vi "ICM Play Back.vi"() -> ()   [LabVIEW 2024]
doc: "OSDS Simulator.vi\n\n This VI is used to produce simulated data streams, either by playing back files recorded with the OSDS Recorder.vi or by creating simulated data consistent with an OSDS definition file.\n\nOCC Streaming Data System Version 1.2.1\nMay, 2015 Original Code Consulting David Thomson\n www.originalcode.com\n\nOSDS is licensed under the Creative Commons Attribution-Share Alike 3.0 license (http://creativecommons.org/). Derivative and commercial works incorporating OSDS are allowed, as long as changes you make are made available to the community at large. Please submit improvements as well as new OSDS Format Files and OSDS Stream Files to support@originalcode.com"
uses:
  ICM Simulator State.ctl
  MICAS-X/Resources/OSDS/OSDS Subvis/OSDS Simulated Channel.ctl
  Bus/Bus.lvclass
  SubVIs/ICM Editor Stop.vi
  Instance           1 22Saved   OSDS Simulator .vi
panel:
  in  "stop":bool
  in  "Tab":enum32{"Setup", "Play Back"}(tab)
  in  "Play Back":bool
  in  "Load":bool
  in  "Loop":bool
  out "Stream File":path
  out "Data":T1(array[cluster]) {"Time Stamp" format="%<%H:%M:%S%1u>t"}
  in  "Display Style":enum16{"Normal", "Codes", "Password", "Hex"}(ring)
  in  "Clear Error":bool
  in  "Stop Streaming":bool
  out "Error":errorcluster
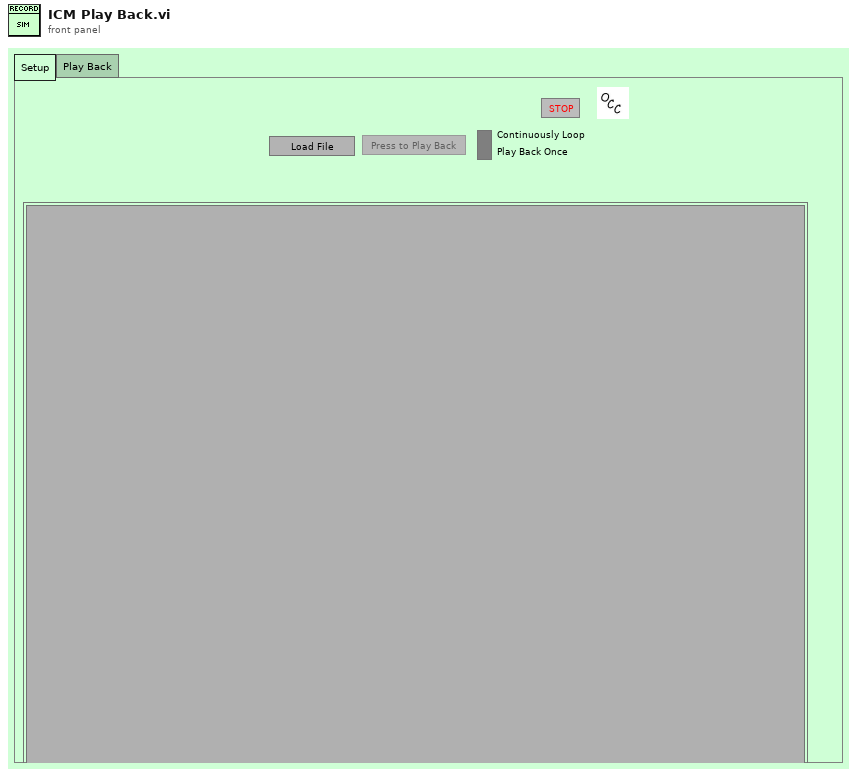
[diagram p1: front panel]
types:
  T1 = cluster{"Time Stamp":dbl, "Length":i32, "Data":string}[]
  T2 = typedef "ICM Simulator State.ctl" = enum16{"Initialize", "Wait", "Open File", "Open ICM", "Write String", "Stop Streaming", "Stop"}
  T3 = enum32{"invalid app kind", "Development System", "Run Time System", "Student Edition", "Embedded LabVIEW", "Evaluation", "Custom"}
  T4 = enum8{"Enabled", "Disabled", "Disabled and Grayed Out"}
  T5 = typedef "OSDS Simulated Channel.ctl" = enum16{"Zero", "Second", "Minute", "Hour", "Day", "Month", "Year", "Day of Year", "Sec of Day", "Latitude", "Longitude", "Altitude", "Nan", "Count", "Random", "One"}
  T6 = cluster{"Streaming?":bool, "Start Time":timestamp, "Current Position":i32, "Handle Out":variant, "Simulated Channels":T5[]}
  T7 = cluster{"Time Stamp":dbl, "Length":i32, "Data":string}
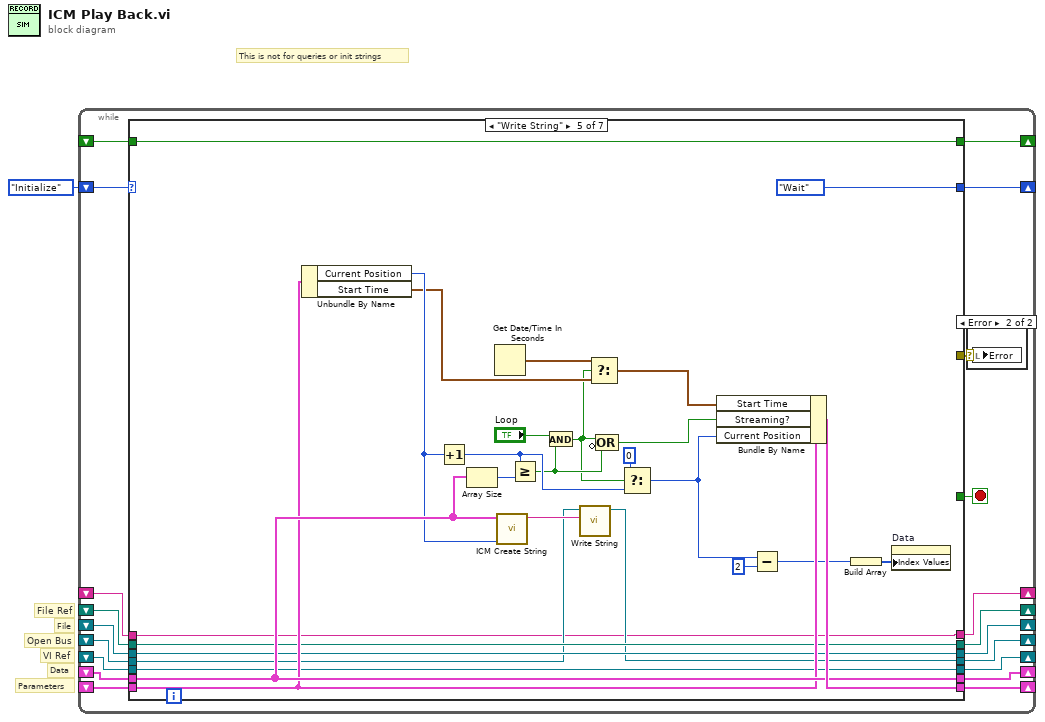
[diagram p0: block diagram]
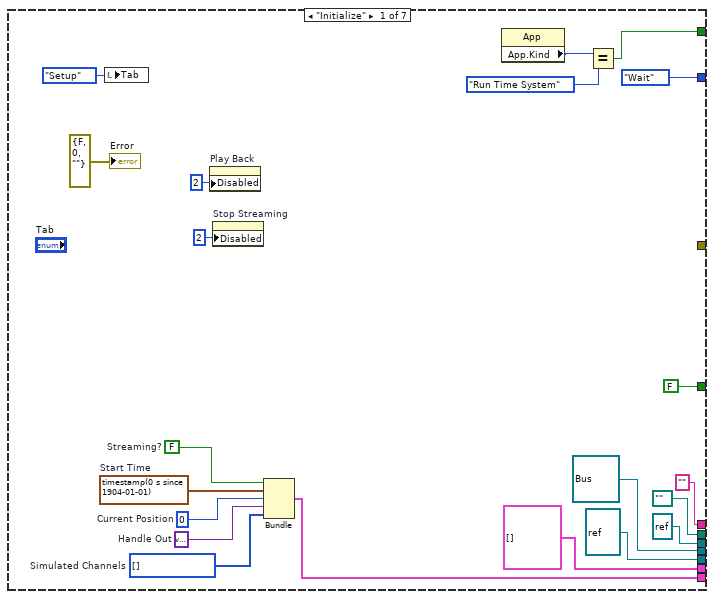
[diagram p2: hidden frame]
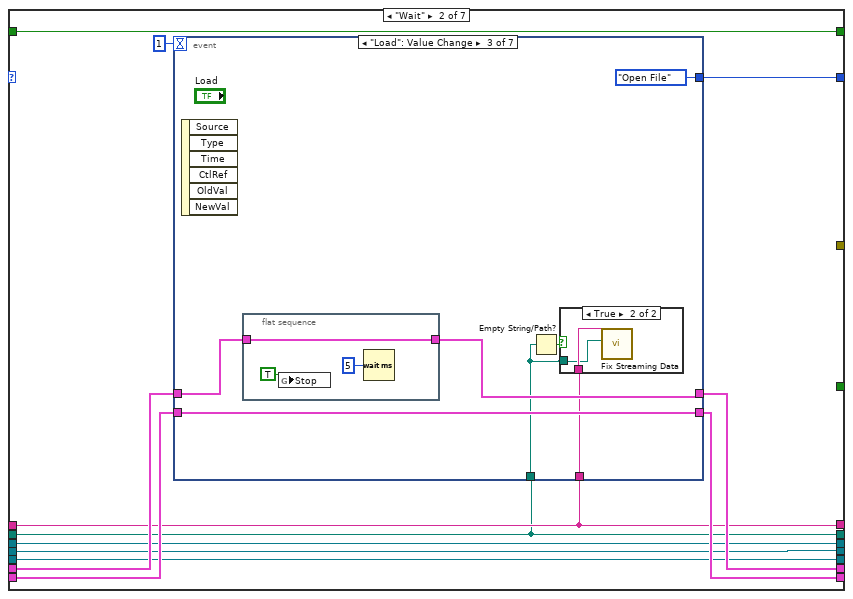
[diagram p3: hidden frame]
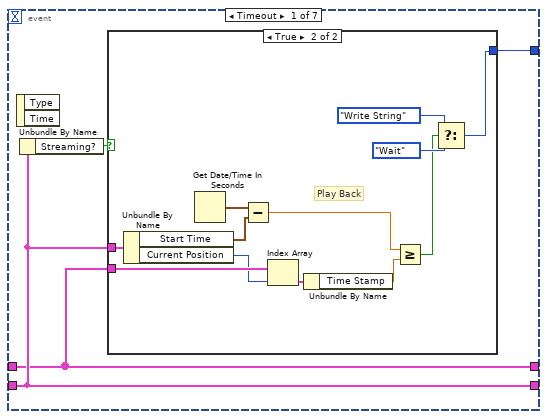
[diagram p4: hidden frame]
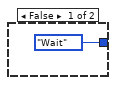
[diagram p5: hidden frame]
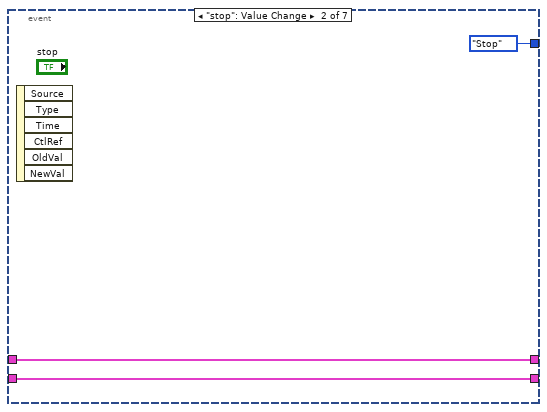
[diagram p6: hidden frame]
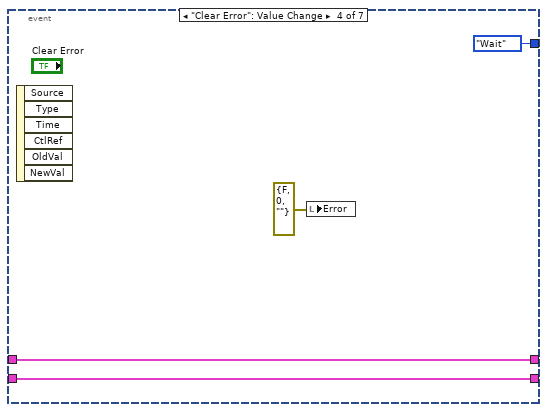
[diagram p8: hidden frame]
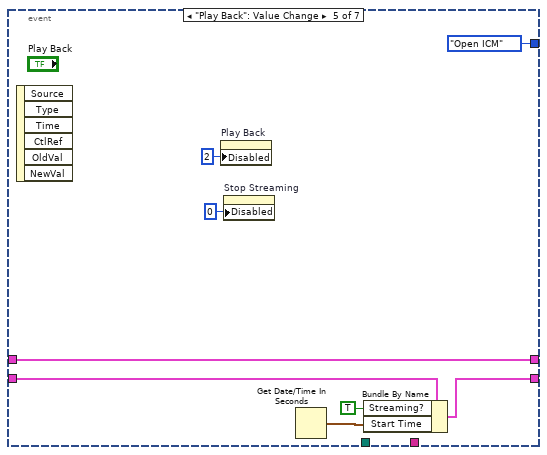
[diagram p9: hidden frame]
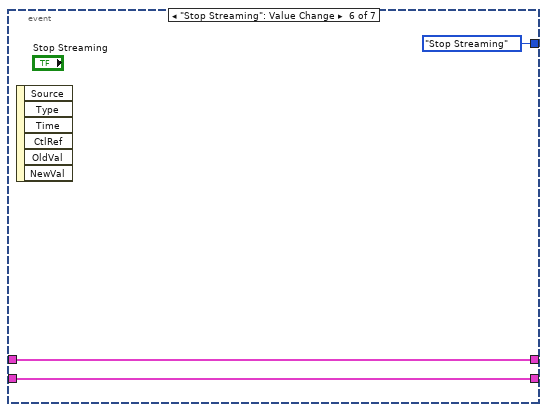
[diagram p10: hidden frame]
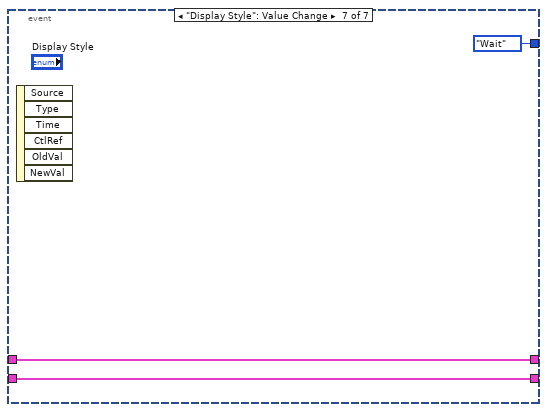
[diagram p11: hidden frame]
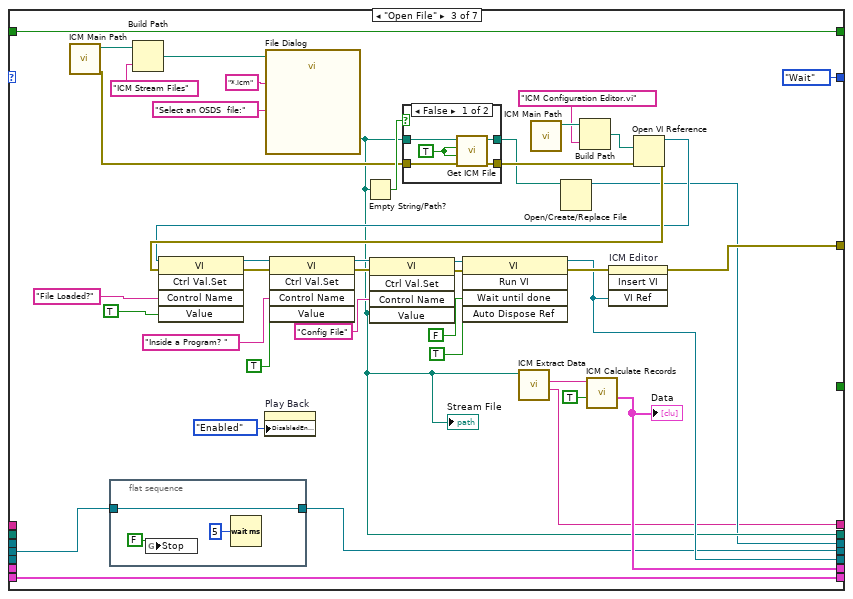
[diagram p12: hidden frame]
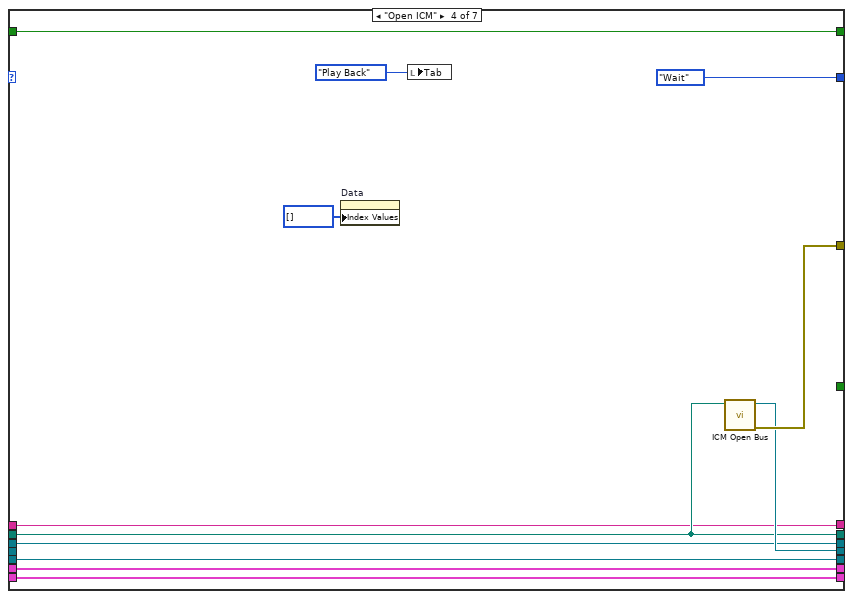
[diagram p14: hidden frame]
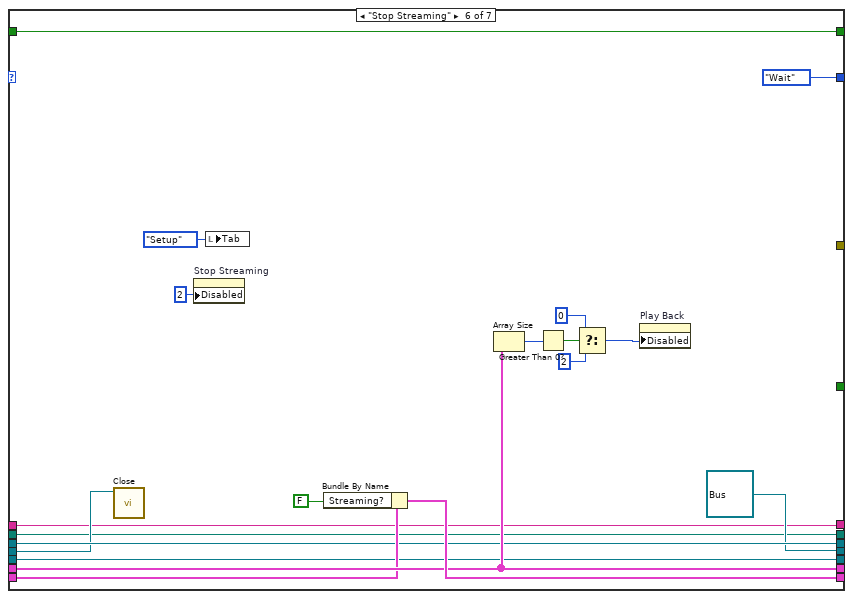
[diagram p15: hidden frame]
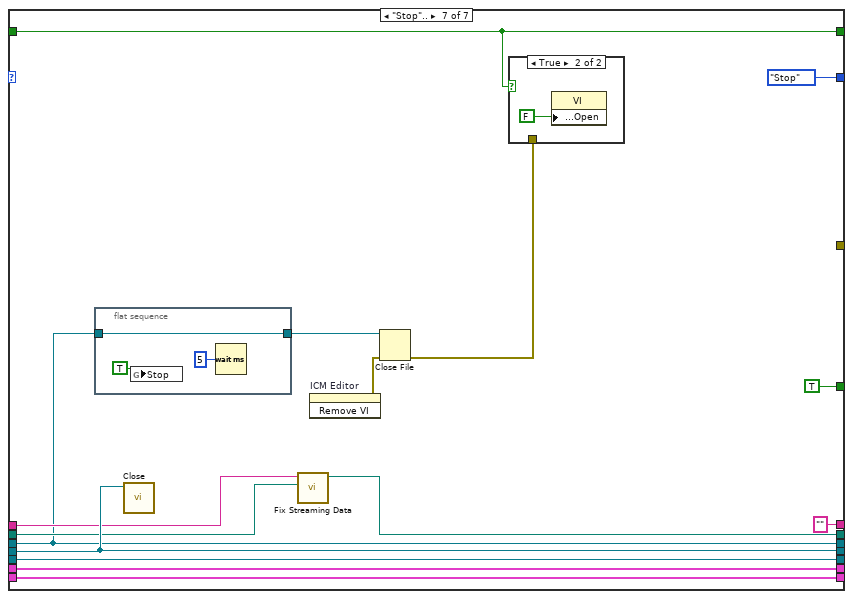
[diagram p16: hidden frame]
diagram:
  # "File Ref"
  # "This is not for queries or init strings"
  # "File"
  # "Open Bus"
  # "VI Ref"
  # "Parameters"
  # "Data"
  n1 = while {
    shift-right: [w21] -> _
    shift-left: ICM_Simulator_State."Initialize" ("Simulator State") -> [w6]
    shift-right: [w18] -> _
    shift-left: _ -> [w17]
    shift-right: [w16] -> _
    shift-left: _ -> [w15]
    shift-right: [w14] -> _
    shift-left: _ -> [w13]
    shift-right: [w12] -> _
    shift-left: _ -> [w10]
    shift-right: [w9] -> _
    shift-left: _ -> [w8]
    shift-right: [w11] -> _
    shift-left: _ -> [w7]
    shift-right: [w5] -> _
    shift-left: _ -> [w4]
    shift-right: [w3] -> _
    shift-left: _ -> [w2]
    stop <- w20 stop-if-true
    n2 = case shown="\"Write String\"" w6 {
      tunnel: [ICM_Simulator_State."Wait" ("Simulator State") w53 ICM_Simulator_State."Wait" ("Simulator State") ICM_Simulator_State."Wait" ("Simulator State") ICM_Simulator_State."Wait" ("Simulator State") ICM_Simulator_State."Wait" ("Simulator State") ICM_Simulator_State."Stop" ("Simulator State")] -> w21
      tunnel: [FALSE _ _ _ _ _ TRUE] -> w20
      tunnel: [_ _ w115 w163 _ _ _] -> w19
      tunnel: [T1 [] ("Data") w51 w110 w167 w191 w205 w227] -> w18
      tunnel: w17 -> [_ w52 _ w167 w191 w205 w227]
      tunnel: [w26 w49 w118 w165 w192 w206 w226] -> w16
      tunnel: w15 -> [_ w50 w118 w165 w189 w203 w226]
      tunnel: [w29 w48 w141 w166 w171 w202 w225] -> w14
      tunnel: w13 -> [_ w48 w141 w166 w171 w202 w225]
      tunnel: [refnum<vi> refnum ("vi reference") w47 w114 w164 w184 w201 w223] -> w12
      tunnel: [refnum<class "Bus.lvclass"> refnum ("Bus Out") w46 w105 w162 w179 refnum<class "Bus.lvclass"> refnum ("Bus out") w224] -> w11
      tunnel: w10 -> [_ w47 _ w164 w184 w201 w223]
      tunnel: [refnum<file> refnum ("refnum out") w44 w108 w161 w183 w200 w217] -> w9
      tunnel: w8 -> [_ w44 _ w161 w183 w200 w217]
      tunnel: w7 -> [_ w46 w106 _ w178 w199 w224]
      tunnel: [path "" ("selected path") w43 w109 w160 w182 w197 w221] -> w5
      tunnel: w4 -> [_ w43 _ w160 w182 w197 w220]
      tunnel: ["" ("Stream Data with Separator") w45 w107 w157 w169 w196 "" ("Stream Data with Separator")] -> w3
      tunnel: w2 -> [_ w45 _ w157 w169 w196 w218]
      frame "Initialize" {
        w32 = T5[] [] items=["Zero", "Second", "Minute", "Hour", "Day", "Month", "Year", "Day of Year", "Sec of Day", "Latitude", "Longitude", "Altitude", "Nan", "Count", "Random", "One"]  # Simulated Channels
        w37 = variant  # Handle Out
        w39 = timestamp(0 s since 1904-01-01)  # Start Time
        w35 = FALSE  # Streaming?
        w38 = 0  # Current Position
        n3 = local write "Tab"(enum32{"Setup", "Play Back"}."Setup" ("Tab")) -> ()
        n4 = property on="Play Back" class="Bool"("Disabled"=u8 2) -> ()  [unwired: 2 in, 2 out]
        n5 = property on="Stop Streaming" class="Bool"("Disabled"=u8 2) -> ()  [unwired: 2 in, 2 out]
        n6 = Bundle("Streaming?"=w35, "Start Time"=w39, "Current Position"=w38, "Handle Out"=w37, "Simulated Channels"=w32) -> (w26:T6)  [unwired: 1 in]
        n7 = property class="App"() -> ("App.Kind"=w31:T3)  [unwired: 2 in, 2 out]
        n8 = Equal?(x=w31, y=T3."Run Time System") -> (x = y?=w29:bool)
        "Error" <- errorcluster {"status"=FALSE, "code"=0, "source"=""} ("Error")
      }
      frame "Wait" {
        n9 = event shown="[2] \"Load\": Value Change" {
          selector: _ -> [_ _ _ _ _ _ _]
          dyn-events: _ -> [_ _ _ _ _ _ _]
          timeout: 1 -> [_ _ _ _ _ _ _]
          tunnel: [w57 ICM_Simulator_State."Stop" ("Simulator State") ICM_Simulator_State."Open File" ("Simulator State") ICM_Simulator_State."Wait" ("Simulator State") ICM_Simulator_State."Open ICM" ("Simulator State") ICM_Simulator_State."Stop Streaming" ("Simulator State") ICM_Simulator_State."Wait" ("Simulator State")] -> w53
          tunnel: w52 -> [w55 w73 w79 w90 w98 w100 w103]
          tunnel: [w55 w73 w78 w90 w98 w100 w103] -> w51
          tunnel: [w56 w72 w80 w87 w95 w99 w102] -> w49
          tunnel: w50 -> [w56 w72 w80 w87 w96 w99 w102]
          tunnel: w45 -> [_ _ w76 _ _ _ _]
          tunnel: w43 -> [_ _ w75 _ _ _ _]
          event Timeout {
            n10 = event-data() -> ()  [unwired: 1 in, 2 out]
            n11 = Unbundle By Name(w56) -> ("Streaming?"=w58:bool)
            n12 = case shown="True" w58 {
              tunnel: [ICM_Simulator_State."Wait" ("Simulator State") w65] -> w57
              tunnel: w56 -> [_ w70]
              tunnel: w55 -> [_ w68]
              frame False {
              }
              frame True {
                # "Play Back"
                n13 = Unbundle By Name(w70) -> ("Start Time"=w69:timestamp, "Current Position"=w66:i32)
                n14 = Get Date/Time In Seconds() -> (seconds since 1Jan1904=w71:timestamp)
                n15 = Subtract(x=w71, y=w69) -> (x-y=w67:dbl)
                n16 = Index Array(array=w68, index=w66) -> (element=w61:T7)
                n17 = Unbundle By Name(w61) -> ("Time Stamp"=w60:dbl)
                n18 = Greater Or Equal?(x=w67, y=w60) -> (x >= y?=w62:bool)
                n19 = Select(t=ICM_Simulator_State."Write String" ("Simulator State"), s=w62, f=ICM_Simulator_State."Wait" ("Simulator State")) -> (s? t:f=w65:T2)
              }
            }
          }
          event "stop": Value Change {
            n20 = event-data() -> ()  [unwired: 1 in, 6 out]
          }
          event "Load": Value Change {
            n21 = event-data() -> ()  [unwired: 1 in, 6 out]
            n22 = flat-sequence {
              tunnel: w79 -> [w84]
              tunnel: [w84] -> w78
              frame #0 {
                n23 = global write "ICM Editor Stop.vi" "Stop"(TRUE ("Stop")) -> ()
                n24 = Wait (ms)(milliseconds to wait=u32 5) -> ()  [unwired: 1 out]
              }
            }
            n25 = Empty String/Path?(string/path=w75) -> (empty?=w77:bool)
            n26 = case shown="True" w77 {
              tunnel: w76 -> [_ w83]
              tunnel: w75 -> [_ w82]
              frame False {
              }
              frame True {
                n27 = call "Fix Streaming Data.vi"("ICM File In"=w82, "Data String"=w83) -> ()  [unwired: 8 in, 2 out]
              }
            }
          }
          event "Clear Error": Value Change {
            n28 = event-data() -> ()  [unwired: 1 in, 6 out]
            n29 = local write "Error"(errorcluster {"status"=FALSE, "code"=0, "source"=""} ("Error")) -> ()
          }
          event "Play Back": Value Change {
            n30 = event-data() -> ()  [unwired: 1 in, 6 out]
            n31 = property on="Play Back" class="Bool"("Disabled"=u8 2) -> ()  [unwired: 2 in, 2 out]
            n32 = property on="Stop Streaming" class="Bool"("Disabled"=u8 0) -> ()  [unwired: 2 in, 2 out]
            n33 = Get Date/Time In Seconds() -> (seconds since 1Jan1904=w91:timestamp)
            n34 = Bundle By Name(cluster=w96, "Streaming?"=TRUE ("Simulate?"), "Start Time"=w91) -> (w95:T6)
          }
          event "Stop Streaming": Value Change {
            n35 = event-data() -> ()  [unwired: 1 in, 6 out]
          }
          event "Display Style": Value Change {
            n36 = event-data() -> ()  [unwired: 1 in, 6 out]
          }
        }
      }
      frame "Open File" {
        n37 = call "ICM Main Path.vi"() -> ("error out"=w119:errorcluster, "ICM Root Path"=w140:path)  [unwired: 9 in, 1 out]
        n38 = flat-sequence {
          tunnel: [w147] -> w105
          tunnel: w106 -> [w147]
          frame #0 {
            n39 = global write "ICM Editor Stop.vi" "Stop"(FALSE ("Stop")) -> ()
            n40 = Wait (ms)(milliseconds to wait=u32 5) -> ()  [unwired: 1 out]
          }
        }
        n41 = Build Path(base path=w140, name or relative path="ICM Stream Files") -> (appended path=w142:path)
        n42 = property on="Play Back" class="Bool"("DisabledEnum"=T4."Enabled" ("Disabled")) -> ()  [unwired: 2 in, 2 out]
        n43 = call "File Dialog"("start path"=w142, "prompt"="Select an OSDS  file:", "pattern (all files)"="*.icm") -> ("selected path"=w109:path)  [unwired: 9 in, 3 out]
        "Stream File" <- w109
        n44 = Empty String/Path?(string/path=w109) -> (empty?=w133:bool)
        n45 = case shown="False" w133 {
          tunnel: w109 -> [w154 w155]
          tunnel: [w152 w156] -> w137
          tunnel: w119 -> [w151 w156]
          tunnel: [w150 w155] -> w117
          frame False {
            w153 = TRUE ("Allow New?")
            n46 = call "Get ICM File.vi"("error in (no error)"=w151, "Re-Init?"=w153, "Allow New?"=w153, "ICM File In"=w154) -> ("error out"=w152:errorcluster, "ICM File"=w150:path)  [unwired: 6 in]
          }
          frame True {
          }
        }
        n47 = call "ICM Extract Data.vi"("Stream File"=w109) -> ("Stream Data with Separator"=w107:string, "Stream Data"=w113:string)  [unwired: 7 in, 2 out]
        n48 = call "ICM Main Path.vi"() -> ("ICM Root Path"=w138:path)  [unwired: 9 in, 2 out]
        n49 = Open/Create/Replace File(file path (use dialog)=w117) -> (refnum out=w108:refnum<file>)  [unwired: 5 in, 2 out]
        n50 = Build Path(base path=w138, name or relative path="ICM Configuration Editor.vi") -> (appended path=w139:path)
        n51 = call "ICM Calculate Records.vi"("Assemble?"=TRUE, "Stream Data"=w113) -> ("Data"=w110:T1)  [unwired: 8 in, 1 out]
        "Data" <- w110
        n52 = Open VI Reference(vi path=w139, error in (no error)=w137) -> (vi reference=w135:refnum<vi>, error out=w136:errorcluster)  [unwired: 4 in]
        n53 = invoke class="VI" method="Ctrl Val.Set"(reference=w135, error in=w136, "Control Name"="File Loaded?", "Value"=TRUE ("Allow New?")) -> (reference out=w125:refnum<vi>, error out=w134:errorcluster)  [unwired: 1 in, 3 out]
        n54 = invoke class="VI" method="Ctrl Val.Set"(reference=w125, error in=w134, "Control Name"="Inside a Program? ", "Value"=TRUE ("Allow New?")) -> (reference out=w122:refnum<vi>, error out=w121:errorcluster)  [unwired: 1 in, 3 out]
        n55 = invoke class="VI" method="Ctrl Val.Set"(reference=w122, error in=w121, "Control Name"="Config File", "Value"=w109) -> (reference out=w124:refnum<vi>, error out=w123:errorcluster)  [unwired: 1 in, 3 out]
        n56 = invoke class="VI" method="Run VI"(reference=w124, error in=w123, "Wait until done"=FALSE ("Wait Until Done"), "Auto Dispose Ref"=TRUE ("Auto Dispose Reference")) -> (reference out=w114:refnum<vi>, error out=w116:errorcluster)  [unwired: 1 in, 3 out]
        n57 = invoke on="ICM Editor" class="SubPnl" method="Insert VI"(error in=w116, "VI Ref"=w114) -> (error out=w115:errorcluster)  [unwired: 2 in, 3 out]
      }
      frame "Open ICM" {
        n58 = property on="Data" class="Arr (strict)"("Index Values"=u32[] []) -> ()  [unwired: 2 in, 2 out]
        n59 = local write "Tab"(enum32{"Setup", "Play Back"}."Play Back" ("Tab")) -> ()
        n60 = call "ICM Open Bus.vi"("ICM File In"=w160) -> ("error out"=w163:errorcluster, "Bus out"=w162:refnum<class "Bus.lvclass">)  [unwired: 9 in]
      }
      frame "Write String" {
        n61 = Unbundle By Name(w189) -> ("Current Position"=w190:i32, "Start Time"=w188:timestamp)
        n62 = Increment(x=w190) -> (x+1=w194:i32)
        n63 = Array Size(array=w191) -> (size(s)=w177:i32)
        n64 = Get Date/Time In Seconds() -> (seconds since 1Jan1904=w172:timestamp)
        n65 = call "ICM Create String.vi"("Data"=w191, "Current Position"=w190) -> ("String Out"=w180:string)  [unwired: 8 in]
        n66 = Greater Or Equal?(x=w194, y=w177) -> (x >= y?=w175:bool)
        n67 = And(x="Loop", y=w175) -> (x .and. y?=w173:bool)
        n68 = call-dynamic "Write String.vi"("String"=w180, "Bus in"=w178) -> ("Bus out"=w179:refnum<class "Bus.lvclass">)  [unwired: 8 in, 1 out]
        n69 = Select(t=w172, s=w173, f=w188) -> (s? t:f=w187:timestamp)
        n70 = Compound Arithmetic op=OR(w173, invert w175) -> (w193:bool)
        n71 = Select(t=0, s=w173, f=w194) -> (s? t:f=w186:i32)
        n72 = Bundle By Name(cluster=w189, "Start Time"=w187, "Streaming?"=w193, "Current Position"=w186) -> (w192:T6)
        n73 = Subtract(x=w186, y=2) -> (x-y=w170:i32)
        n74 = Build Array(w170) -> (w181:i32[])
        n75 = property on="Data" class="Arr (strict)"("Index Values"=w181) -> ()  [unwired: 2 in, 2 out]
      }
      frame "Stop Streaming" {
        n76 = call-dynamic "Close.vi"("Bus in"=w199) -> ()  [unwired: 9 in, 2 out]
        n77 = property on="Stop Streaming" class="Bool"("Disabled"=u8 2) -> ()  [unwired: 2 in, 2 out]
        n78 = local write "Tab"(enum32{"Setup", "Play Back"}."Setup" ("Tab")) -> ()
        n79 = Bundle By Name(cluster=w203, "Streaming?"=FALSE) -> (w206:T6)
        n80 = Array Size(array=w205) -> (size(s)=w211:i32)
        n81 = Greater Than 0?(x=w211) -> (x > 0?=w210:bool)
        n82 = Select(t=u8 0 ("Disabled"), s=w210, f=u8 2 ("Disabled")) -> (s? t:f=w204:u8)
        n83 = property on="Play Back" class="Bool"("Disabled"=w204) -> ()  [unwired: 2 in, 2 out]
      }
      frame "Stop".. {
        n84 = flat-sequence {
          tunnel: w217 -> [w230]
          tunnel: [w230] -> w216
          frame #0 {
            n85 = global write "ICM Editor Stop.vi" "Stop"(TRUE ("Stop")) -> ()
            n86 = Wait (ms)(milliseconds to wait=u32 5) -> ()  [unwired: 1 out]
          }
        }
        n87 = call-dynamic "Close.vi"("Bus in"=w224) -> ()  [unwired: 9 in, 2 out]
        n88 = call "Fix Streaming Data.vi"("ICM File In"=w220, "Data String"=w218) -> ("path"=w221:path)  [unwired: 8 in, 1 out]
        n89 = invoke on="ICM Editor" class="SubPnl" method="Remove VI"() -> (error out=w222:errorcluster)  [unwired: 3 in, 2 out]
        n90 = Close File(refnum=w216, error in=w222) -> (error out=w215:errorcluster)  [unwired: 1 out]
        n91 = case shown="True" w225 {
          tunnel: w215 -> [_ _]
          frame False {
          }
          frame True {
            n92 = property class="VI"("Front Panel.Open"=FALSE ("Front Panel Window:Open")) -> ()  [unwired: 2 in, 2 out]
          }
        }
      }
    }
    n93 = case shown="Error" w19 {
      selector: w19 -> [_ w234]
      frame No Error {
      }
      frame Error {
        n94 = local write "Error"(w234) -> ()
      }
    }
  }
